vi "Super Market Billing System edit 3.vi"() -> ()   [LabVIEW 2021]
panel:
  in  "Tab Control":enum32{"Page 1", "Page 2"}(tab)
  out "Horizontal Progress Bar":u8(slide) scale=0.0..100.0
  in  "Refresh Button":bool
  in  "Password":string
  in  "System Login":string
  in  "stop":bool
  out "Bill":dbl
  out "discount":string
  out "Price per 1kg":dbl
  out "price 4":dbl
  out "price 3":dbl
  out "price 2":dbl
  out "Vegetables":dbl
  in  "Carrot":bool
  in  "quantity 5":dbl
  in  "Cabege":bool
  in  "quantity 4":dbl
  in  "Bringle":bool
  in  "quantity 3":dbl
  in  "Beans":bool
  in  "quantity 2":dbl
  in  "Leeks":bool
  in  "Quantities":dbl
  out "Total Bill":dbl
  in  "Banana":bool
  out "Fruits":dbl
  in  "Apple":bool
  out "price 6":dbl
  in  "quantity 6":dbl
  in  "Orange":bool
  out "price 7":dbl
  in  "quantity 7":dbl
  in  "Graps":bool
  out "price 8":dbl
  in  "quantity 8":dbl
  in  "Papaya":bool
  in  "quantity 9":dbl
  out "Price per 1kg 2":dbl
  in  "Quantities 2":dbl
  in  "Rise 5Kg":bool
  in  "Dal 1Kg":bool
  in  "Salt 400g":bool
  in  "Coconut Oil 1L":bool
  in  "Cilli Powder 100g":bool
  in  "Curry Powder 100g":bool
  in  "Turmeric Powder 50g":bool
  in  "Milk Powder 1kg":bool
  in  "Sugar  1kg":bool
  out "price 10":dbl
  out "price 5":dbl
  out "price 9":dbl
  out "price 11":dbl
  in  "quantity 14":dbl
  out "price 12":dbl
  in  "quantity 15":dbl
  out "price 13":dbl
  in  "quantity 16":dbl
  out "Price per 1kg 4":dbl
  in  "quantity 13":dbl
  in  "Quantities 4":dbl
  in  "quantity 12":dbl
  in  "quantity 11":dbl
  in  "quantity 10":dbl
  in  "Tea 100g":bool
  in  "Quantities":dbl
  in  "quantity 17":dbl
  out "Product List":dbl
  out "?":dbl
  out "Price":dbl
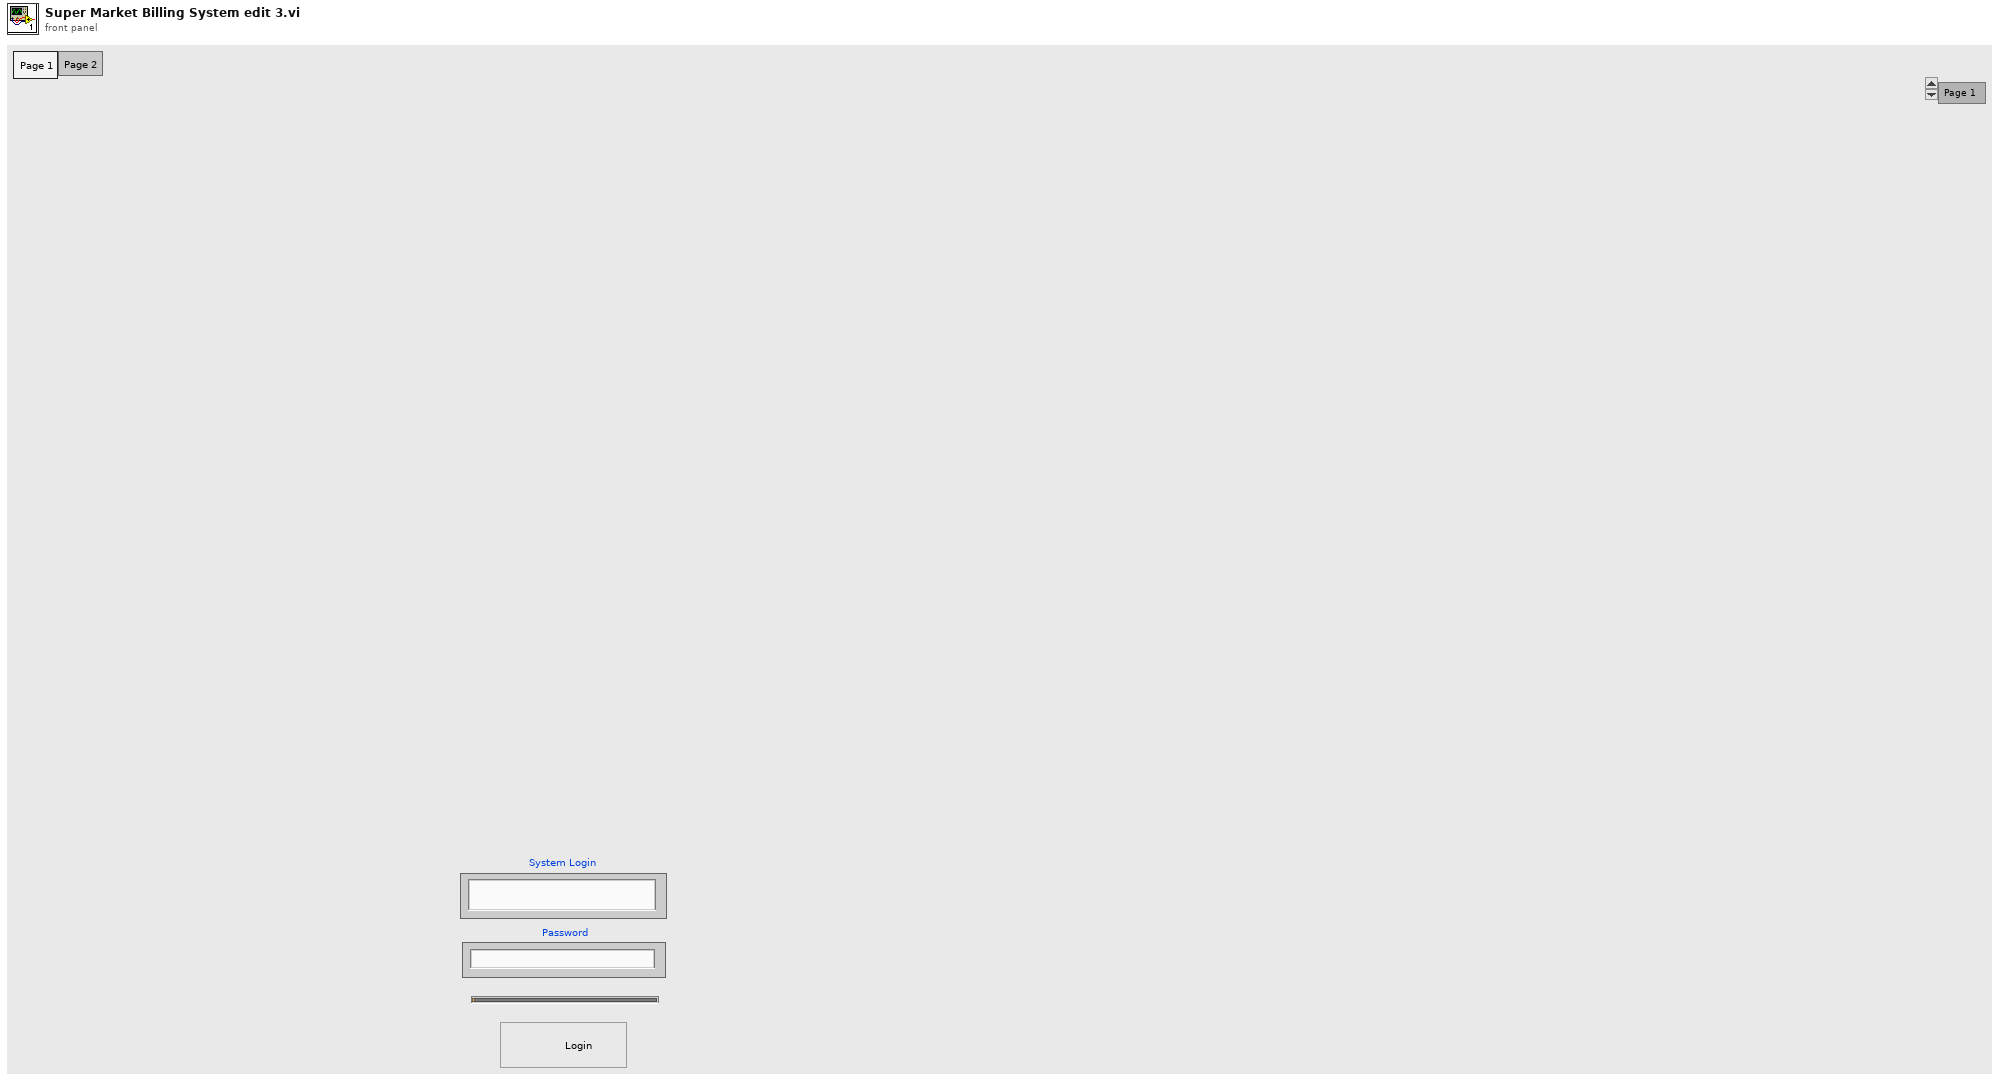
[diagram p1: front panel]
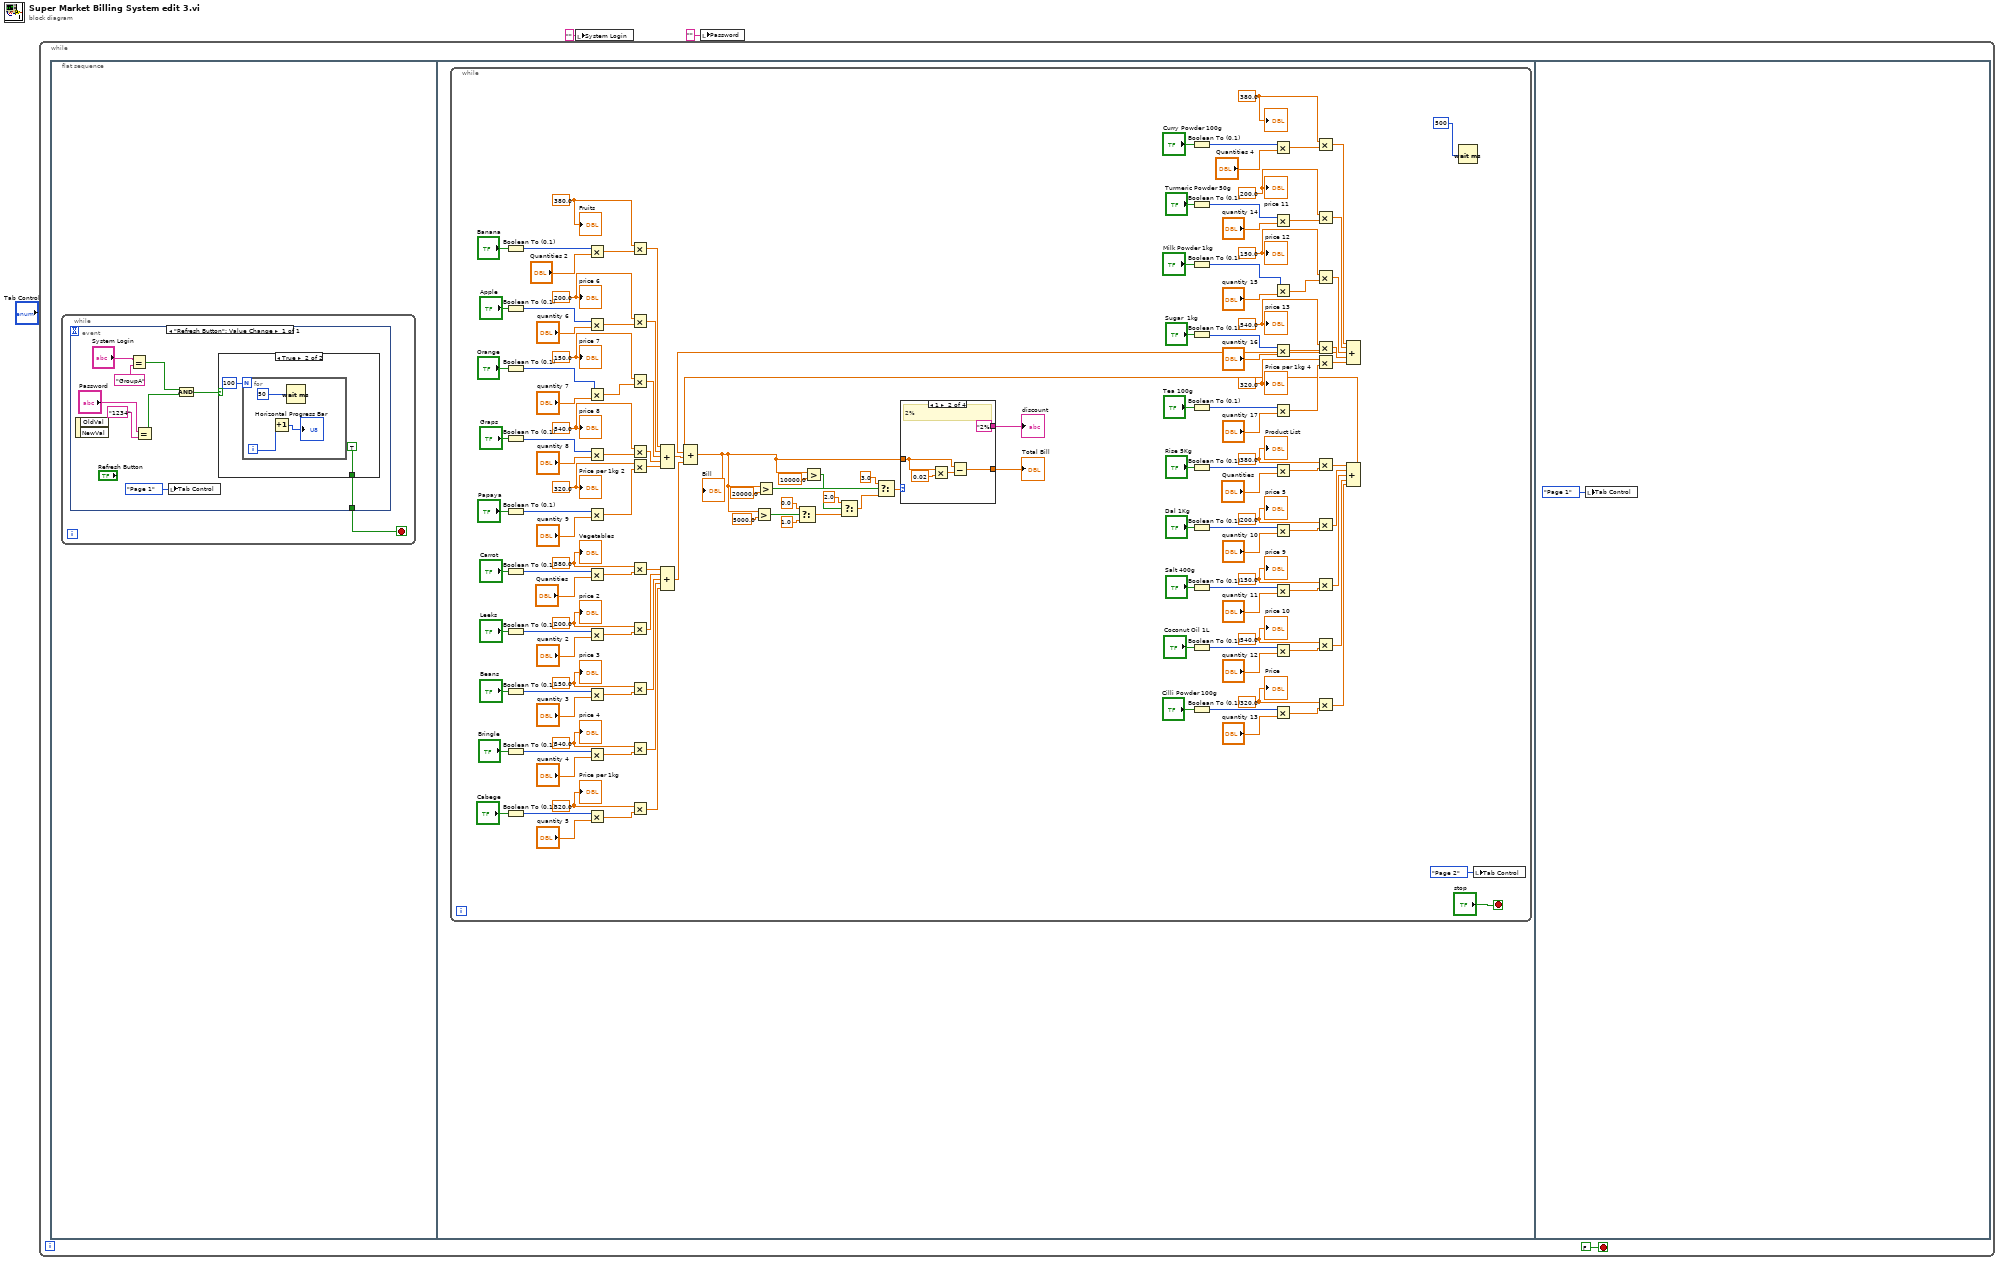
[diagram p0: block diagram]
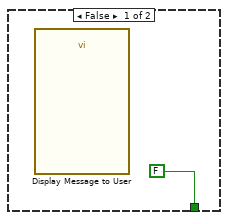
[diagram p2: hidden frame]
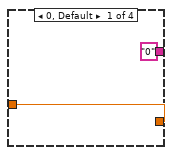
[diagram p3: hidden frame]
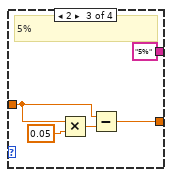
[diagram p4: hidden frame]
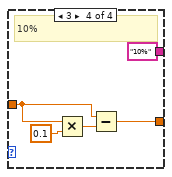
[diagram p5: hidden frame]
diagram:
  n1 = while {
    stop <- FALSE stop-if-true
    n2 = flat-sequence {
      frame #0 {
        n3 = while {
          stop <- w4 stop-if-true
          n4 = event shown="[0] \"Refresh Button\": Value Change" {
            selector: _ -> [_]
            dyn-events: _ -> [_]
            timeout: _ -> [_]
            tunnel: [w6] -> w4
            event "Refresh Button": Value Change {
              n5 = event-data() -> ()  [unwired: 1 in, 2 out]
              n6 = Equal?(x="System Login", y="GroupA") -> (x = y?=w9:bool)
              n7 = Equal?(x="Password", y="1234") -> (x = y?=w8:bool)
              n8 = local write "Tab Control"(enum32{"Page 1", "Page 2"}."Page 1" ("Tab Control")) -> ()
              n9 = And(x=w9, y=w8) -> (x .and. y?=w7:bool)
              n10 = case shown="True" w7 {
                tunnel: [FALSE TRUE] -> w6
                frame False {
                  n11 = call "Display Message to User"() -> ()  [unwired: 10 in, 2 out]
                }
                frame True {
                  n12 = for {
                    N: 100 -> [_]
                    i -> [w17]
                    n13 = Increment(x=w17) -> (x+1=→"Horizontal Progress Bar":i32)
                    n14 = Wait (ms)(milliseconds to wait=u32 50 ("millisecond timer value")) -> ()  [unwired: 1 out]
                  }
                }
              }
            }
          }
        }
      }
      frame #1 {
        n15 = while {
          stop <- "stop" stop-if-true
          w125 = 320.0 ("price")
          w118 = 540.0 ("price")
          w115 = 150.0 ("price")
          w108 = 200.0 ("price")
          w105 = 380.0 ("price")
          w155 = 320.0 ("price")
          w148 = 540.0 ("price")
          w145 = 150.0 ("price")
          w138 = 200.0 ("price")
          w135 = 380.0 ("price")
          w48 = 320.0 ("price")
          w41 = 540.0 ("price")
          w38 = 150.0 ("price")
          w31 = 200.0 ("price")
          w28 = 380.0 ("price")
          w78 = 320.0 ("price")
          w71 = 540.0 ("price")
          w68 = 150.0 ("price")
          w61 = 200.0 ("price")
          w58 = 380.0 ("price")
          n16 = Boolean To (0,1)(Boolean="Banana") -> (0, 1=w26:i16)
          n17 = Boolean To (0,1)(Boolean="Apple") -> (0, 1=w33:i16)
          n18 = Boolean To (0,1)(Boolean="Orange") -> (0, 1=w36:i16)
          n19 = Boolean To (0,1)(Boolean="Graps") -> (0, 1=w43:i16)
          n20 = Boolean To (0,1)(Boolean="Papaya") -> (0, 1=w46:i16)
          n21 = Boolean To (0,1)(Boolean="Carrot") -> (0, 1=w56:i16)
          n22 = Boolean To (0,1)(Boolean="Leeks") -> (0, 1=w63:i16)
          n23 = Boolean To (0,1)(Boolean="Beans") -> (0, 1=w66:i16)
          n24 = Boolean To (0,1)(Boolean="Bringle") -> (0, 1=w73:i16)
          n25 = Boolean To (0,1)(Boolean="Cabege") -> (0, 1=w76:i16)
          n26 = Multiply(x=w26, y="Quantities 2") -> (x*y=w29:dbl)
          n27 = Multiply(x=w33, y="quantity 6") -> (x*y=w30:dbl)
          n28 = Multiply(x=w36, y="quantity 7") -> (x*y=w39:dbl)
          n29 = Multiply(x=w43, y="quantity 8") -> (x*y=w40:dbl)
          n30 = Multiply(x=w46, y="quantity 9") -> (x*y=w49:dbl)
          n31 = Multiply(x=w56, y="Quantities") -> (x*y=w59:dbl)
          n32 = Multiply(x=w63, y="quantity 2") -> (x*y=w60:dbl)
          n33 = Multiply(x=w66, y="quantity 3") -> (x*y=w69:dbl)
          n34 = Multiply(x=w73, y="quantity 4") -> (x*y=w70:dbl)
          n35 = Multiply(x=w76, y="quantity 5") -> (x*y=w79:dbl)
          n36 = Multiply(x=w28, y=w29) -> (x*y=w50:dbl)
          n37 = Multiply(x=w31, y=w30) -> (x*y=w51:dbl)
          n38 = Multiply(x=w38, y=w39) -> (x*y=w52:dbl)
          n39 = Multiply(x=w41, y=w40) -> (x*y=w53:dbl)
          n40 = Multiply(x=w48, y=w49) -> (x*y=w54:dbl)
          n41 = Multiply(x=w58, y=w59) -> (x*y=w80:dbl)
          n42 = Multiply(x=w61, y=w60) -> (x*y=w81:dbl)
          n43 = Multiply(x=w68, y=w69) -> (x*y=w82:dbl)
          n44 = Multiply(x=w71, y=w70) -> (x*y=w83:dbl)
          n45 = Multiply(x=w78, y=w79) -> (x*y=w84:dbl)
          n46 = Compound Arithmetic op=ADD(w50, w51, w52, w53, w54) -> (w23:dbl)
          n47 = Compound Arithmetic op=ADD(w80, w81, w82, w83, w84) -> (w24:dbl)
          n48 = Boolean To (0,1)(Boolean="Curry Powder 100g") -> (0, 1=w103:i16)
          n49 = Boolean To (0,1)(Boolean="Turmeric Powder 50g") -> (0, 1=w110:i16)
          n50 = Boolean To (0,1)(Boolean="Milk Powder 1kg") -> (0, 1=w113:i16)
          n51 = Boolean To (0,1)(Boolean="Sugar  1kg") -> (0, 1=w120:i16)
          n52 = Boolean To (0,1)(Boolean="Tea 100g") -> (0, 1=w123:i16)
          n53 = Boolean To (0,1)(Boolean="Rise 5Kg") -> (0, 1=w133:i16)
          n54 = Boolean To (0,1)(Boolean="Dal 1Kg") -> (0, 1=w140:i16)
          n55 = Boolean To (0,1)(Boolean="Salt 400g") -> (0, 1=w143:i16)
          n56 = Boolean To (0,1)(Boolean="Coconut Oil 1L") -> (0, 1=w150:i16)
          n57 = Boolean To (0,1)(Boolean="Cilli Powder 100g") -> (0, 1=w153:i16)
          n58 = Multiply(x=w103, y="Quantities 4") -> (x*y=w106:dbl)
          n59 = Multiply(x=w110, y="quantity 14") -> (x*y=w107:dbl)
          n60 = Multiply(x=w113, y="quantity 15") -> (x*y=w116:dbl)
          n61 = Multiply(x=w120, y="quantity 16") -> (x*y=w117:dbl)
          n62 = Multiply(x=w123, y="quantity 17") -> (x*y=w126:dbl)
          n63 = Multiply(x=w133, y="Quantities") -> (x*y=w136:dbl)
          n64 = Multiply(x=w140, y="quantity 10") -> (x*y=w137:dbl)
          n65 = Multiply(x=w143, y="quantity 11") -> (x*y=w146:dbl)
          n66 = Multiply(x=w150, y="quantity 12") -> (x*y=w147:dbl)
          n67 = Multiply(x=w153, y="quantity 13") -> (x*y=w156:dbl)
          n68 = Multiply(x=w105, y=w106) -> (x*y=w127:dbl)
          n69 = Multiply(x=w108, y=w107) -> (x*y=w128:dbl)
          n70 = Multiply(x=w115, y=w116) -> (x*y=w129:dbl)
          n71 = Multiply(x=w118, y=w117) -> (x*y=w130:dbl)
          n72 = Multiply(x=w125, y=w126) -> (x*y=w131:dbl)
          n73 = Multiply(x=w135, y=w136) -> (x*y=w157:dbl)
          n74 = Multiply(x=w138, y=w137) -> (x*y=w158:dbl)
          n75 = Multiply(x=w145, y=w146) -> (x*y=w159:dbl)
          n76 = Multiply(x=w148, y=w147) -> (x*y=w160:dbl)
          n77 = Multiply(x=w155, y=w156) -> (x*y=w161:dbl)
          n78 = Compound Arithmetic op=ADD(w127, w128, w129, w130, w131) -> (w21:dbl)
          n79 = Compound Arithmetic op=ADD(w157, w158, w159, w160, w161) -> (w20:dbl)
          n80 = Compound Arithmetic op=ADD(w20, w21, w23, w24) -> (w22:dbl)
          "Bill" <- w22
          n81 = Greater?(x=w22, y=5000.0) -> (0:w96:bool)
          n82 = Greater?(x=w22, y=20000.0) -> (0:w98:bool)
          n83 = Select(t=0.0, s=w96, f=1.0) -> (s? t:f=w92:dbl)
          n84 = Greater?(x=w22, y=10000.0) -> (0:w97:bool)
          n85 = Select(t=2.0, s=w97, f=w92) -> (s? t:f=w93:dbl)
          n86 = Select(t=3.0, s=w98, f=w93) -> (s? t:f=w94:dbl)
          n87 = case shown="1" w94 {
            tunnel: [w164 w168 w171 w176] -> w99
            tunnel: w22 -> [w164 w166 w172 w177]
            tunnel: ["0" ("discount") "2%" ("discount") "5%" ("discount") "10%" ("discount")] -> w95
            frame 0, Default {
            }
            frame 1 {
              # "2%"
              n88 = Multiply(x=w166, y=0.02) -> (x*y=w167:dbl)
              n89 = Subtract(x=w166, y=w167) -> (x-y=w168:dbl)
            }
            frame 2 {
              # "5%"
              n90 = Multiply(x=w172, y=0.05) -> (x*y=w173:dbl)
              n91 = Subtract(x=w172, y=w173) -> (x-y=w171:dbl)
            }
            frame 3 {
              # "10%"
              n92 = Multiply(x=w177, y=0.1) -> (x*y=w178:dbl)
              n93 = Subtract(x=w177, y=w178) -> (x-y=w176:dbl)
            }
          }
          "Total Bill" <- w99
          "discount" <- w95
          n94 = Wait (ms)(milliseconds to wait=u32 500) -> ()  [unwired: 1 out]
          n95 = local write "Tab Control"(enum32{"Page 1", "Page 2"}."Page 2" ("Tab Control")) -> ()
          "Vegetables" <- w58
          "price 2" <- w61
          "price 3" <- w68
          "price 4" <- w71
          "Price per 1kg" <- w78
          "Fruits" <- w28
          "price 6" <- w31
          "price 7" <- w38
          "price 8" <- w41
          "Price per 1kg 2" <- w48
          "Product List" <- w135
          "price 5" <- w138
          "price 9" <- w145
          "price 10" <- w148
          "Price" <- w155
          "?" <- w105
          "price 11" <- w108
          "price 12" <- w115
          "price 13" <- w118
          "Price per 1kg 4" <- w125
        }
      }
      frame #2 {
        n96 = local write "Tab Control"(enum32{"Page 1", "Page 2"}."Page 1" ("Tab Control")) -> ()
      }
    }
  }
  n97 = local write "System Login"("" ("User Name")) -> ()
  n98 = local write "Password"("" ("Password")) -> ()
